vi "Add Buffer Channels.vi"(4 "channels":T1[](array[typedef]) {"string offset" format="%d bytes"}, 5 "engine (T) / string (F)":bool, 6 "Decimation":u64, 7 "Transfer Group Status":refnum<class "Status.lvclass">, 8 "error in (no error)":errorcluster, 9 "Buffer":refnum<class "Buffer.lvclass">, 10 "parent tag":string, 11 "Application Data In":T4) -> (0 "error out":errorcluster, 3 "Application Data out":T4)   [LabVIEW 2017, in "DSF Core.lvlib"]
uses:
  DSF Core.lvlib
  Main VI/Application Data.ctl
  <vilib>/NI/Memory Manager/Classes/Pointer/Pointer.lvclass
  Classes/Framework/Framework.lvclass
  Buffer Reader/Buffer Data.ctl
  Classes/Buffer/Buffer.lvclass
  C:/Program Files (x86)/National Instruments/LabVIEW 2017/vi.lib/NI/Memory Manager/Classes/Pointer/Pointer.lvclass
  Classes/Transfer Group Status/Status.lvclass
  Typedefs/DSF Data Type.ctl
  Typedefs/DSF Engine Framework Configuration.ctl
  Typedefs/DSF Engine Plugin Configuration.ctl
  Typedefs/DSF Timing Info.ctl
  Typedefs/DSF Engine Plugin Thread Configuration.ctl
  Typedefs/DSF Settings Info.ctl
  Typedefs/DSF Engine Transfer Group Configuration.ctl
  Typedefs/DSF Direction.ctl
  Typedefs/DSF Engine Transfer Configuration.ctl
  Typedefs/DSF Byte Order.ctl
  Typedefs/DSF Engine Channel Configuration.ctl
  Typedefs/DSF Timeout Behavior.ctl
  ID to Tree Items/Tree Item Type.ctl
  <vilib>/NI/Memory Manager/Classes/Pointer/Pointer.lvclass/Pointer.ctl
  Classes/Buffer/Get Buffer Size.vi
  <vilib>/NI/Memory Manager/Classes/Pointer/Get Size.vi
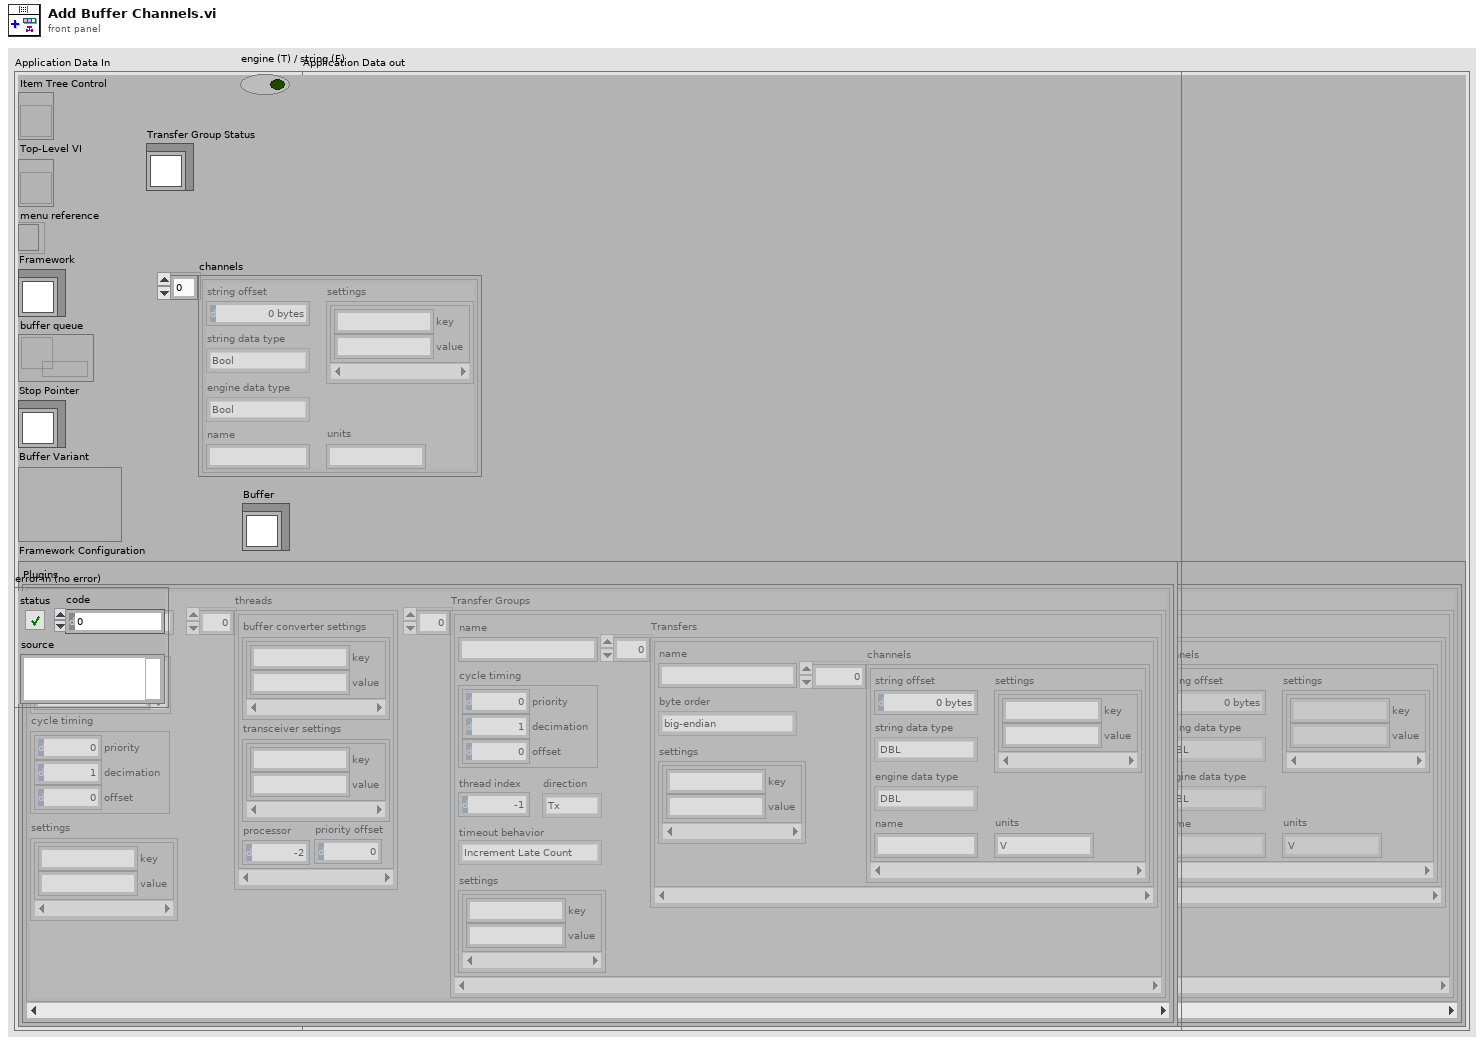
[diagram p1: front panel]
types:
  T1 = typedef "DSF Core.lvlib/DSF Engine Channel Configuration.ctl" = cluster{"string offset":u64, "string data type":T2, "engine data type":T2, "name":string, "settings":T3, "units":string}
  T2 = typedef "DSF Core.lvlib/DSF Data Type.ctl" = enum8{"Bool", "SGL", "DBL", "I8", "I16", "I32", "I64", "U8", "U16", "U32", "U64"}
  T3 = typedef "DSF Core.lvlib/DSF Settings Info.ctl" = cluster{"key":string, "value":string}[]
  T4 = typedef "DSF Core.lvlib/Application Data.ctl" = cluster{"Item Tree Control":refnum<vi>, "Top-Level VI":refnum<vi>, "menu reference":refnum<k9>, "Framework":refnum<class "Framework.lvclass">, "buffer queue":refnum<queue>, "Stop Pointer":refnum<class "Pointer.lvclass">, "Buffer Variant":variant, "Framework Configuration":T5}
  T5 = typedef "DSF Core.lvlib/DSF Engine Framework Configuration.ctl" = cluster{"Plugins":T6[]}
  T6 = typedef "DSF Core.lvlib/DSF Engine Plugin Configuration.ctl" = cluster{"name":string, "components":string[], "cycle timing":T7, "threads":T8[], "Transfer Groups":T9[], "settings":T3}
  T7 = typedef "DSF Core.lvlib/DSF Timing Info.ctl" = cluster{"priority":u64, "decimation":u64, "offset":u64}
  T8 = typedef "DSF Core.lvlib/DSF Engine Plugin Thread Configuration.ctl" = cluster{"buffer converter settings":T3, "transceiver settings":T3, "processor":i32, "priority offset":i16}
  T9 = typedef "DSF Core.lvlib/DSF Engine Transfer Group Configuration.ctl" = cluster{"name":string, "direction":T10, "cycle timing":T7, "thread index":i32, "settings":T3, "Transfers":T11[], "timeout behavior":T13}
  T10 = typedef "DSF Core.lvlib/DSF Direction.ctl" = enum8{"Tx", "Rx"}
  T11 = typedef "DSF Core.lvlib/DSF Engine Transfer Configuration.ctl" = cluster{"name":string, "byte order":T12, "settings":T3, "channels":T1[]}
  T12 = typedef "DSF Core.lvlib/DSF Byte Order.ctl" = enum8{"big-endian", "little-endian"}
  T13 = typedef "DSF Core.lvlib/DSF Timeout Behavior.ctl" = enum8{"Increment Late Count", "Throw Error"}
  T14 = typedef "DSF Core.lvlib/Buffer Data.ctl" = cluster{"Buffer":refnum<class "Buffer.lvclass">, "Status":refnum<class "Status.lvclass">, "decimation":u64, "avg bandwidth":dbl, "data type":T2, "units":string}
  T15 = typedef "DSF Core.lvlib/Tree Item Type.ctl" = enum16{"Framework", "Plugin Group", "Plugin", "Group", "Transfer", "Buffer", "Channel"}
  T16 = typedef "DSF Core.lvlib/Tree Item.ctl" = cluster{"Left Cell String":string, "Child Text":string[], "Child Tag":string, "Glyph Index":i32}
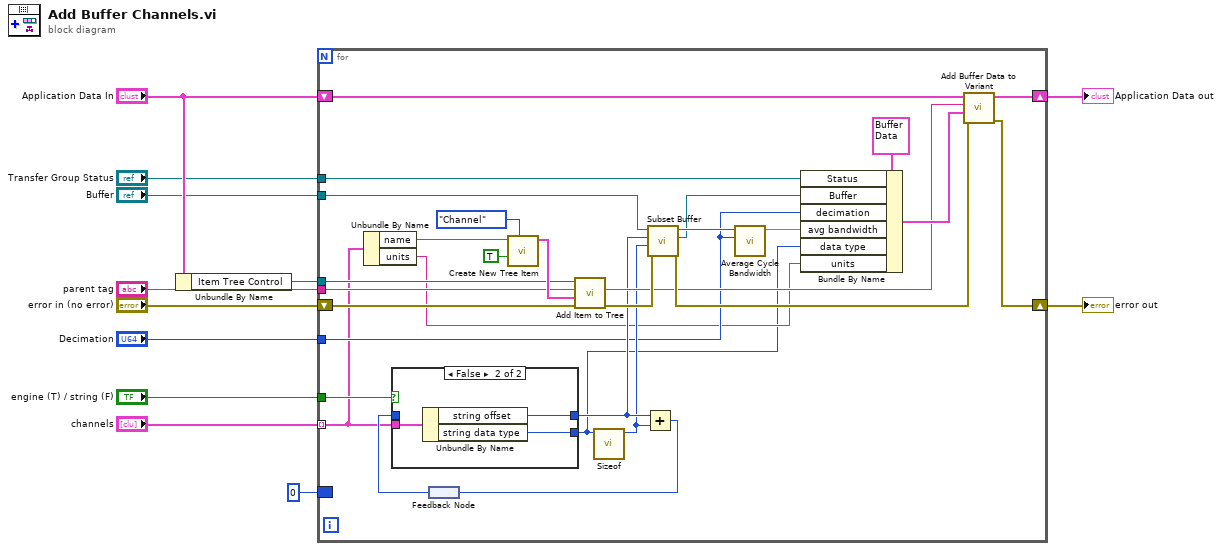
[diagram p0: block diagram]
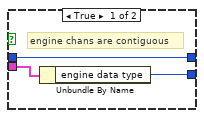
[diagram p2: hidden frame]
diagram:
  n1 = Unbundle By Name("Application Data In") -> ("Item Tree Control"=w8:refnum<vi>)
  n2 = for {
    tunnel: w8 -> [w32]
    tunnel: "parent tag" -> [w31]
    tunnel: "Transfer Group Status" -> [w30]
    tunnel: "Buffer" -> [w15]
    tunnel: "Decimation" -> [w18]
    shift-right: [w40] -> w11
    shift-left: "error in (no error)" -> [w37]
    shift-right: [w41] -> w12
    shift-left: "Application Data In" -> [w33]
    tunnel: "channels" -> [w17] mode=indexing
    tunnel: "engine (T) / string (F)" -> [w26]
    border: u64 0 -> [_]
    n3 = Unbundle By Name(w17) -> ("name"=w16:string, "units"=w14:string)
    n4 = feedback #1() -> (w25:u64)
    n5 = case shown="False" w26 {
      tunnel: w17 -> [w44 w47]
      tunnel: [w43 w46] -> w13
      tunnel: [w42 w45] -> w20
      tunnel: w25 -> [w42 _]
      frame True {
        # "engine chans are contiguous"
        n6 = Unbundle By Name(w44) -> ("engine data type"=w43:T2)
      }
      frame False {
        n7 = Unbundle By Name(w47) -> ("string offset"=w45:u64, "string data type"=w46:T2)
      }
    }
    n8 = call "Create New Tree Item.vi"("Item Type"=Tree_Item_Type."Channel", "found?"=TRUE, "Left Cell String"=w16) -> ("Item"=w34:T16)  [unwired: 7 in, 1 out]
    n9 = call "Add Item to Tree.vi"("error in (no error)"=w37, "Item"=w34, "parent tag"=w31, "TreeControl in"=w32) -> ("error out"=w23:errorcluster, "new item tag"=w21:string)  [unwired: 5 in, 1 out]
    n10 = call "Sizeof.vi"("data type"=w13) -> ("size in bytes"=w19:u64)  [unwired: 9 in, 1 out]
    n11 = Add(x=w20, y=w19) -> (x+y=w24:u64)
    n12 = feedback-in #1(w24) -> ()
    n13 = call "Subset Buffer.vi"("error in (no error)"=w23, "size"=w19, "offset"=w20, "Buffer in"=w15) -> ("error out"=w22:errorcluster, "subset Buffer"=w27:refnum<class "Buffer.lvclass">, "Buffer out"=w28:refnum<class "Buffer.lvclass">)  [unwired: 4 in, 1 out]
    n14 = call "Average Cycle Bandwidth.vi"("Decimation"=w18, "Buffer"=w28) -> ("avergage cycle bandwidth"=w29:dbl)  [unwired: 9 in]
    n15 = Bundle By Name(cluster=T14 {"Buffer"=refnum, "Status"=refnum, "decimation"=0, "avg bandwidth"=0.0, "data type"=enum."Bool", "units"=""} ("Buffer data"), "Status"=w30, "Buffer"=w27, "decimation"=w18, "avg bandwidth"=w29, "data type"=w13, "units"=w14) -> (w39:T14)
    n16 = call "Add Buffer Data to Variant.vi"("error in (no error)"=w22, "Buffer data"=w39, "tag"=w21, "Application Data In in"=w33) -> ("error out"=w40:errorcluster, "Application Data In out"=w41:T4)  [unwired: 6 in]
  }
  "error out" <- w11
  "Application Data out" <- w12
